vi "Read.vi"(8 "error in (no error)":errorcluster, 11 "ClientUI in":refnum<class "ClientUI.lvclass">) -> (0 "error out":errorcluster, 2 "Message":string, 3 "ClientUI out":refnum<class "ClientUI.lvclass">)   [LabVIEW 2018, in "ClientUI.lvlib" / "ClientUI.lvclass"]
uses:
  ClientUI.lvclass
  ClientUI.lvclass/ClientUI.ctl
  TCP_Client/TCP_Client/TCP_Client.lvclass
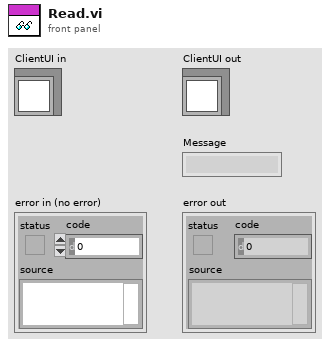
[diagram p1: front panel]
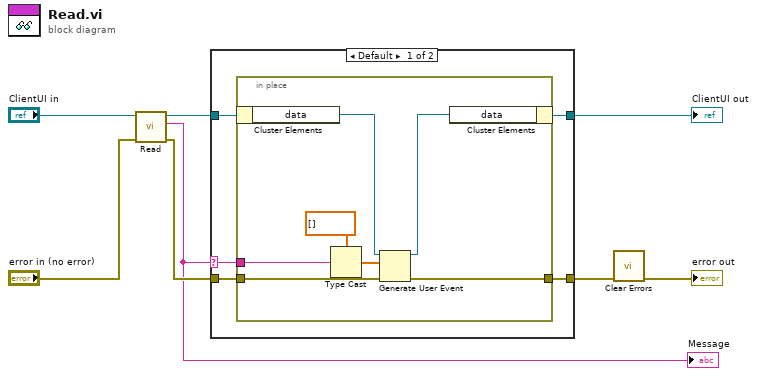
[diagram p0: block diagram]
diagram:
  n1 = call-parent "Read.vi"("error in (no error)"="error in (no error)", "TCP_Client in"="ClientUI in") -> ("error out"=w5:errorcluster, "Message"=w2:string, "TCP_Client out"=w4:refnum<class "ClientUI.lvclass">)  [unwired: 7 in]
  "Message" <- w2
  n2 = case shown="Default" w2 {
    selector: w2 -> [w9 _]
    tunnel: [w13 w21] -> w6
    tunnel: w5 -> [w12 w21]
    tunnel: w4 -> [w11 w22]
    tunnel: [w10 w22] -> w3
    frame Default {
      n3 = in-place {
        in-place-border: [w20] -> w13
        in-place-border: w12 -> [w19]
        in-place-border: w9 -> [w14]
        n4 = in-place-cluster #1(w11) -> ("data"=w18:refnum<user-event>)
        n5 = Type Cast(type=dbl[] [], x=w14) -> (*(type *) &x=w15:dbl[])
        n6 = Generate User Event(user event=w18, event data cluster=w15, error in=w19) -> (user event out=w17:refnum<user-event>, error out=w20:errorcluster)  [unwired: 1 in]
        n7 = in-place-cluster #1("data"=w17) -> (w10:refnum<class "ClientUI.lvclass">)
      }
    }
    frame "" {
    }
  }
  "ClientUI out" <- w3
  n8 = call <vilib>:"Clear Errors.vi"("error in (no error)"=w6) -> ("error out"=→"error out":errorcluster)  [unwired: 5 in, 1 out]
